vi "Get Target IP Address.vi"(8 "error in":errorcluster, 11 "Device Item Ref in":T1 format="%.0x") -> (0 "error out":errorcluster, 2 "IP Address":string, 3 "Device Item Ref out":T1 format="%.0x")   [LabVIEW 2027, in "NIVS Hardware Discovery.lvlib"]
uses:
  NIVS Hardware Discovery.lvlib
  <vilib>/NI VeriStand/Custom Device Tools/Custom Device Utility Library/Custom Device Utility Library.lvlib
  <vilib>/NI VeriStand/Custom Device API/Custom Device API.lvlib
  <vilib>/NI VeriStand/Custom Device API/Custom Device Item Ref.ctl
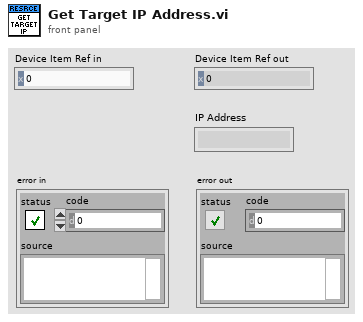
[diagram p1: front panel]
types:
  T1 = typedef "Custom Device API.lvlib/Custom Device Item Ref.ctl" = u64
  T2 = typedef "Custom Device API.lvlib/Custom Device Pointer.ctl" = refnum<k24>
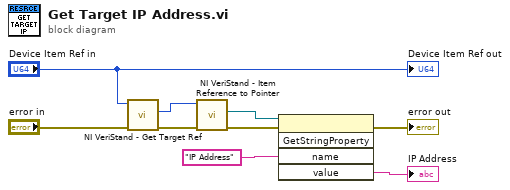
[diagram p0: block diagram]
diagram:
  n1 = call <vilib>:"NI VeriStand - Get Target Ref.vi"("error in"="error in", "Item Ref in"="Device Item Ref in") -> ("error out"=w3:errorcluster, "Target Ref"=w6:T1)  [unwired: 6 in, 2 out]
  n2 = call <vilib>:"NI VeriStand - Item Reference to Pointer.vi"("error in (no error)"=w3, "Item Ref in"=w6) -> ("error out"=w2:errorcluster, "Node Pointer"=w7:T2)  [unwired: 6 in, 2 out]
  n3 = invoke method="GetStringProperty"(reference=w7, error in=w2, "name"="IP Address") -> (error out=→"error out":errorcluster, "value"=→"IP Address":string)  [unwired: 2 in, 3 out]
  "Device Item Ref out" <- "Device Item Ref in"
